vi "Default Settings.vi"() -> (3 "Default Settings":T1={"Calibration Array"=[], "Hardware Config Cluster"=[], "Trigger Settings"={"Trigger Type"=enum."No Trigger", "Digital Start"={"Source"="", "Digital Start Trigger Edge"=0}, "Digital Pause"={"Source"="APFI0", "Digital Pause Trigger Pause When"=10192}, "Digital Reference"={"Source"="", "Digital Start Trigger Edge"=10280, "Digital Reference Pretrigger Samples"=0}, "Analog Start"={"Source"="", "Analog Slope"=10093, "Analog Start Trigger Hysteresis"=0.0, "Analog Start Trigger Level"=0.0}, "Analog Pause"={"Source"="", "Analog Start Trigger Level"=0.0, "Analog Pause Trigger Pause When"=10093}, "Analog Reference"={"Source"="", "Slope"=10280, "Pretrigger Samples"=0, "Level"=0.0}, "Time Start"={"Select Time\nManually"=FALSE, "When"=timestamp(0 s since 1904-01-01)}}, "Log File Base Path"=path "", "DAQmx Timing Settings"={"rate"=1000.0, "source"="OnboardClock", "sample mode"=10178, "samples per channel"=1000}} {"DAQmx Timing Settings"."sample mode" items=["Finite Samples"=10178, "Continuous Samples"=10123, "Hardware Timed Single Point"=12522]; "DAQmx Timing Settings"."rate" format="%0.2f"; "Trigger Settings"."Time Start"."When" format="%<%x %.3X>T"; "Trigger Settings"."Analog Reference"."Level" format="%0.2f"; "Trigger Settings"."Analog Reference"."Slope" items=["Rising"=10280, "Falling"=10171]; "Trigger Settings"."Analog Pause"."Analog Pause Trigger Pause When" items=["Above Level"=10093, "Below Level"=10107]; "Trigger Settings"."Analog Pause"."Analog Start Trigger Level" format="%0.2f"; "Trigger Settings"."Analog Start"."Analog Start Trigger Level" format="%0.2f"; "Trigger Settings"."Analog Start"."Analog Start Trigger Hysteresis" format="%.2f"; "Trigger Settings"."Analog Start"."Analog Slope" items=["Rising"=10280, "Falling"=10171]; "Trigger Settings"."Digital Reference"."Digital Start Trigger Edge" items=["Rising"=10280, "Falling"=10171]; "Trigger Settings"."Digital Pause"."Digital Pause Trigger Pause When" items=["High"=10192, "Low"=10214]; "Trigger Settings"."Digital Start"."Digital Start Trigger Edge" items=["Rising"=10280, "Falling"=10171]; "Hardware Config Cluster"."Unit" items=["Volts", "From Custom Scale"]})   [LabVIEW 2020, in "Settings Editor.lvlib"]
doc: "_____\nBased on DQMH Project Template 6.0.0.91."
uses:
  Settings Editor.lvlib
  Settings--cluster.ctl
  DAQmx Config--cluster.ctl
  DAQmx Trigger Settings--cluster.ctl
  DAQmx Timing--cluster.ctl
  <vilib>/Utility/sysdir.llb/System Directory Type.ctl
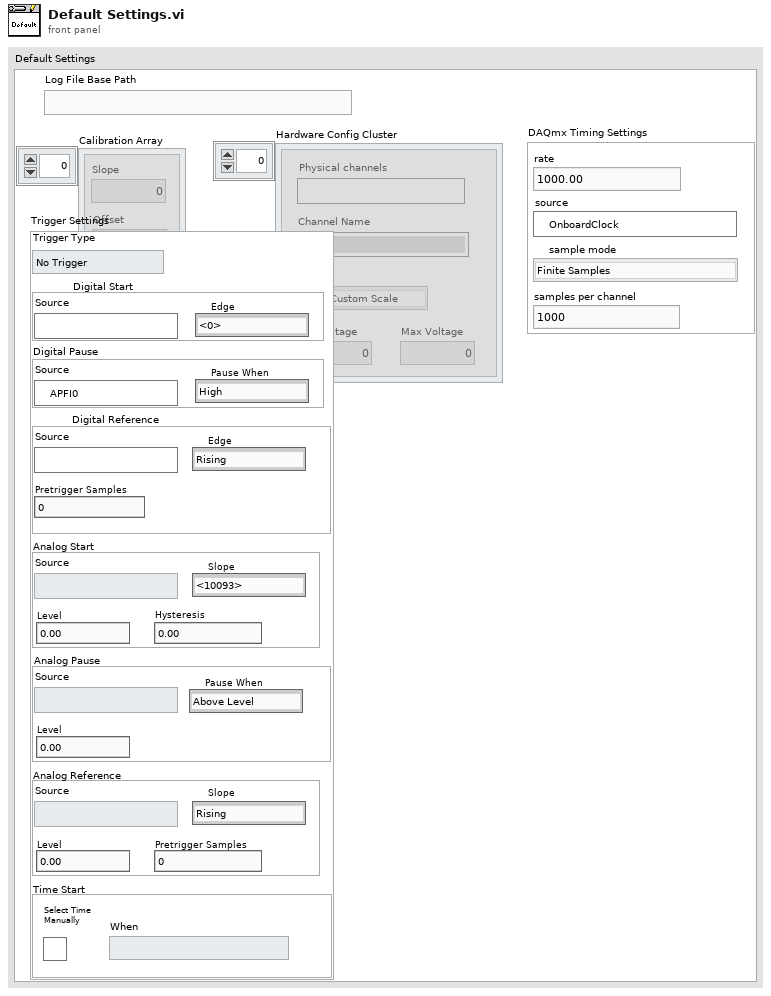
[diagram p1: front panel]
types:
  T1 = typedef "Settings Editor.lvlib/Settings--cluster.ctl" = cluster{"Calibration Array":cluster{"Slope":dbl, "Offset":dbl}[], "Hardware Config Cluster":T2, "Trigger Settings":T3, "Log File Base Path":path, "DAQmx Timing Settings":T4}
  T2 = typedef "Settings Editor.lvlib/DAQmx Config--cluster.ctl" = cluster{"Physical channels":tag, "Channel Name":string, "Unit":i32, "Min Voltage":dbl, "Max Voltage":dbl}[]
  T3 = typedef "Settings Editor.lvlib/DAQmx Trigger Settings--cluster.ctl" = cluster{"Trigger Type":enum32{"No Trigger", "Digital Start", "Digital Pause", "Digital Reference", "Analog Start", "Analog Pause", "Analog Reference", "Time Start"}, "Digital Start":cluster{"Source":tag, "Digital Start Trigger Edge":i32}, "Digital Pause":cluster{"Source":tag, "Digital Pause Trigger Pause When":i32}, "Digital Reference":cluster{"Source":tag, "Digital Start Trigger Edge":i32, "Digital Reference Pretrigger Samples":u32}, "Analog Start":cluster{"Source":string, "Analog Slope":i32, "Analog Start Trigger Hysteresis":dbl, "Analog Start Trigger Level":dbl}, "Analog Pause":cluster{"Source":string, "Analog Start Trigger Level":dbl, "Analog Pause Trigger Pause When":i32}, "Analog Reference":cluster{"Source":string, "Slope":i32, "Pretrigger Samples":u32, "Level":dbl}, "Time Start":cluster{"Select Time\nManually":bool, "When":timestamp}}
  T4 = typedef "Settings Editor.lvlib/DAQmx Timing--cluster.ctl" = cluster{"rate":dbl, "source":tag, "sample mode":i32, "samples per channel":i32}
  T5 = typedef "System Directory Type.ctl" = i32
  T6 = enum32{"No Trigger", "Digital Start", "Digital Pause", "Digital Reference", "Analog Start", "Analog Pause", "Analog Reference", "Time Start"}
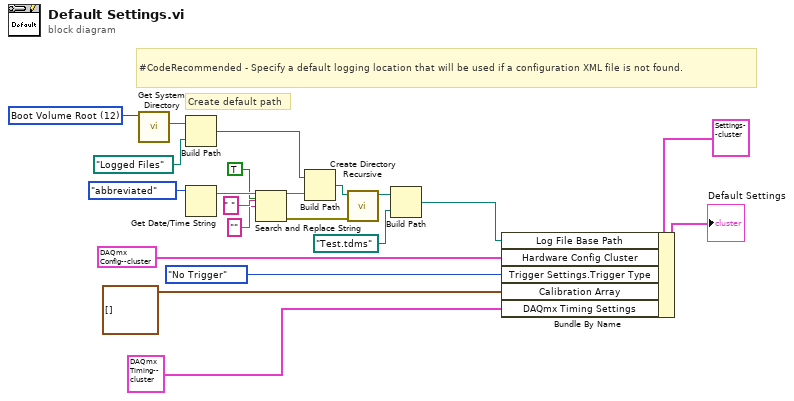
[diagram p0: block diagram]
diagram:
  w16 = T5 12 items=["User Home"=0, "User Desktop"=1, "User Documents"=2, "User Application Data"=3, "User Preferences"=4, "User Temporary"=5, "Public Documents"=6, "Public Application Data"=7, "Public Preferences"=8, "Public Cache"=13, "System Core Libraries"=9, "System Installed Libraries"=10, "Application Files"=11, "Boot Volume Root"=12] ("system directory type")
  # "Create default path"
  # "#CodeRecommended - Specify a default logging location that will be used if a configuration XML file is not found."
  n1 = call <vilib>:"Get System Directory.vi"("system directory type"=w16) -> ("system directory"=w15:path)  [unwired: 10 in]
  n2 = Build Path(base path=w15, name or relative path=path "Logged Files") -> (appended path=w6:path)
  n3 = Get Date/Time String(date format (0)=enum16{"short", "long", "abbreviated"}."abbreviated") -> (date string=w11:string)  [unwired: 2 in, 1 out]
  n4 = Search and Replace String(replace all?=TRUE ("replace all? (F)"), input string=w11, search string=" ", replace string="" ("replace string (\"\")")) -> (result string=w7:string, error out=w4:errorcluster)  [unwired: 4 in, 2 out]
  n5 = Build Path(base path=w6, name or relative path=w7) -> (appended path=w5:path)
  n6 = call <vilib>:"Create Directory Recursive.vi"("error in (no error)"=w4, "directory"=w5) -> ("directory copy"=w14:path)  [unwired: 3 in, 2 out]
  n7 = Build Path(base path=w14, name or relative path=path "Test.tdms") -> (appended path=w3:path)
  n8 = Bundle By Name(cluster=T1 {"Calibration Array"=[{"Slope"=1.0, "Offset"=0.0}], "Hardware Config Cluster"=[], "Trigger Settings"={"Trigger Type"=enum."No Trigger", "Digital Start"={"Source"="", "Digital Start Trigger Edge"=0}, "Digital Pause"={"Source"="APFI0", "Digital Pause Trigger Pause When"=10192}, "Digital Reference"={"Source"="", "Digital Start Trigger Edge"=10280, "Digital Reference Pretrigger Samples"=0}, "Analog Start"={"Source"="", "Analog Slope"=10093, "Analog Start Trigger Hysteresis"=0.0, "Analog Start Trigger Level"=0.0}, "Analog Pause"={"Source"="", "Analog Start Trigger Level"=0.0, "Analog Pause Trigger Pause When"=10093}, "Analog Reference"={"Source"="", "Slope"=10280, "Pretrigger Samples"=0, "Level"=0.0}, "Time Start"={"Select Time\nManually"=FALSE, "When"=timestamp(0 s since 1904-01-01)}}, "Log File Base Path"=path "", "DAQmx Timing Settings"={"rate"=0.0, "source"="", "sample mode"=0, "samples per channel"=0}} ("Default Settings"), "Log File Base Path"=w3, "Hardware Config Cluster"=T2 [{"Physical channels"="Dev1/ai0", "Channel Name"="pd", "Unit"=0, "Min Voltage"=-0.5, "Max Voltage"=0.5}] ("Hardware Config Cluster- Array"), "Trigger Settings.Trigger Type"=T6."No Trigger", "Calibration Array"=cluster{"Slope":dbl, "Offset":dbl}[] [], "DAQmx Timing Settings"=T4 {"rate"=1000.0, "source"="OnboardClock", "sample mode"=10178, "samples per channel"=1000}) -> (→"Default Settings":T1)
